vi "permute_rows.vi"(1 "Array":dbl[][](array[numeric]), 2 "Permutation":i32[](array[numeric])) -> (0 "Result":dbl[][](array[numeric]))   [LabVIEW 2013]
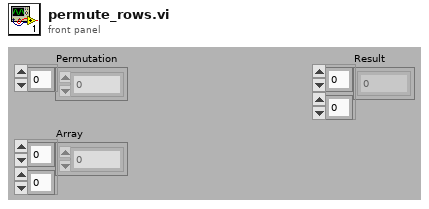
[diagram p1: front panel]
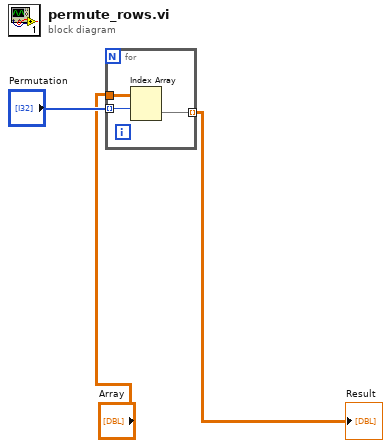
[diagram p0: block diagram]
diagram:
  n1 = for {
    tunnel: "Array" -> [w6]
    tunnel: "Permutation" -> [w5] mode=indexing
    tunnel: [w4] -> w3 mode=indexing
    n2 = Index Array(array=w6, index (row)=w5) -> (element=w4:dbl[])  [unwired: 1 in]
  }
  "Result" <- w3
